vi "FRIC_navX_Util_DecodeProtocol_UInt32.vi"(7 "length":i32=2, 8 "Device Register":T1=18 items=["WHOAMI"=0, "HW_REV"=1, "FW_VER_MAJOR"=2, "FW_VER_MINOR"=3, "UPDATE_RATE_HZ"=4, "ACCEL_FSR_G"=5, "GYRO_FSR_DPS"=6, "OP_STATUS"=8, "CAL_STATUS"=9, "SELFTEST_STATUS"=10, "CAPABILITY_FLAGS_L"=11, "CAPABILITY_FLAGS_H"=12, "SENSOR_STATUS"=16, "TIMESTAMP"=18, "YAW"=22, "ROLL"=24, "PITCH"=26, "HEADING"=28, "FUSED_HEADING"=30, "ALTITUDE_I"=32, "ALTITUDE_D"=34, "LINERA_ACC_X"=36, "LINERA_ACC_Y"=38, "LINERA_ACC_Z"=40, "QUAT_W"=42, "QUAT_X"=44, "QUAT_Y"=46, "QUAT_Z"=48, "MPU_TEMP_C"=50, "GYRO_X"=52, "GYRO_Y"=54, "GYRO_Z"=56, "ACC_X"=58, "ACC_Y"=60, "ACC_Z"=62, "MAG_X"=64, "MAG_Y"=66, "MAG_Z"=68, "PRESSURE_I"=70, "PRESSURE_D"=72, "PRESSURE_TEMP"=74, "YAW_OFFSET"=76, "QUAT_OFFSET_W"=78, "QUAT_OFFSET_X"=80, "QUAT_OFFSET_Y"=82, "QUAT_OFFSET_Z"=84, "INTEGRATION_CONTROL"=86, "VELOCITY_X"=88, "VELOCITY_Y"=92, "VELOCITY_Z"=96, "DISPLACMENT_X"=100, "DISPLACMENT_Y"=104, "DISPLACEMENT_Z"=108]) -> (3 "UInt32":u32)   [LabVIEW 2015, in "navX AE v1.lvlib"]
uses:
  navX Library v2/_TypeDefs/Z900_navX_DeviceRegisters.ctl
  navX AE v1.lvlib
  navX Library v2/navX Library v2.lvlib
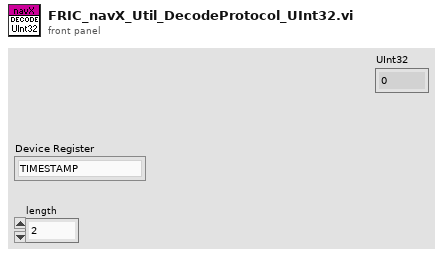
[diagram p1: front panel]
types:
  T1 = typedef "navX Library v2.lvlib/Z900_navX_DeviceRegisters.ctl" = u8
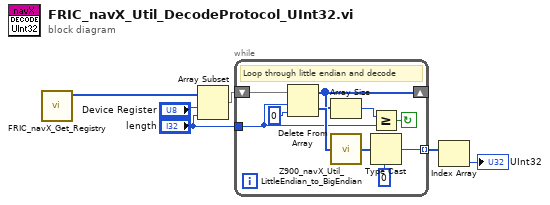
[diagram p0: block diagram]
diagram:
  n1 = call "FRIC_navX_Get_Registry.vi"() -> ("Registry (out)"=w1:u8[])  [unwired: 10 in, 1 out]
  n2 = Array Subset(array=w1, index="Device Register", length="length") -> (w5:u8[])
  n3 = while {
    shift-right: [w10] -> _
    shift-left: w5 -> [w16]
    tunnel: [w11] -> w3 mode=indexing
    tunnel: "length" -> [w7]
    stop <- w8 continue-if-true
    # "Loop through little endian and decode"
    n4 = Delete From Array(array=w16, length=w7, index=0) -> (deleted portion=w12:u8[], array with subset deleted=w10:u8[])
    n5 = Array Size(array=w10) -> (size(s)=w9:i32)
    n6 = call "Z900_navX_Util_LittleEndian_to_BigEndian.vi"("Little Endian"=w12) -> ("Big Endian"=w14:u8[])
    n7 = Greater Or Equal?(x=w9, y=w7) -> (x >= y?=w8:bool)
    n8 = Type Cast(type=u32 0, x=w14) -> (*(type *) &x=w11:u32)
  }
  n9 = Index Array(array=w3) -> (element=→"UInt32":u32)  [unwired: 1 in]
